vi "Get Required Driver Type.vi"(8 "error in (no error)":errorcluster, 11 "Test Instrument Msg in":refnum<class "Test Instrument Msg.lvclass">) -> (0 "error out":errorcluster, 2 "Required Driver Type":refnum<class "Instrument Driver.lvclass">, 3 "Test Instrument Msg out":refnum<class "Test Instrument Msg.lvclass">)   [LabVIEW 2020, in "Test.lvlib" / "Test Instrument Msg.lvclass"]
uses:
  Test Instrument Msg.lvclass
  PPL/HDH.Actor Framework.Core.Instrument Driver.lvlibp/Instrument Driver/Instrument Driver.lvclass
  Instrument/Test Instrument/Test Instrument.lvclass
  C:/Current projects/WS/PPL/HDH.Actor Framework.Core.Instrument Driver.lvlibp/Instrument Driver/Instrument Driver.lvclass
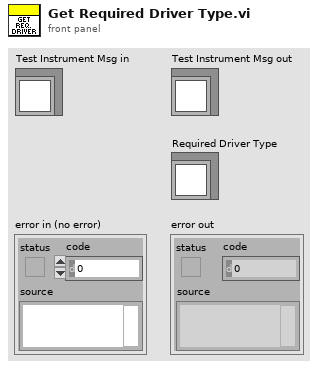
[diagram p1: front panel]
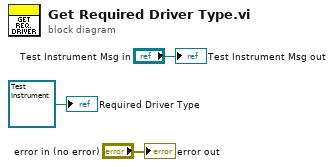
[diagram p0: block diagram]
diagram:
  "error out" <- "error in (no error)"
  "Test Instrument Msg out" <- "Test Instrument Msg in"
  "Required Driver Type" <- refnum<class "Test Instrument.lvclass"> refnum ("Test.lvlib:Test Instrument.lvclass")
